vi "FlatToRichcif_manager_CreatePluginLoaderRequest.vi"(5 "OutputClusterType":T1, 11 "InputCluster":T4) -> (3 "OutputCluster":T1)   [LabVIEW 2021, in "CIF_Manager_client.lvlib"]
uses:
  cif_manager_CreatePluginLoaderRequest_Flat.ctl
  cif_manager_LoaderInfo_Flat.ctl
  cif_manager_LoaderType.ctl
  cif_manager_CreatePluginLoaderRequest.ctl
  cif_manager_LoaderInfo.ctl
  CIF_Manager_client.lvlib
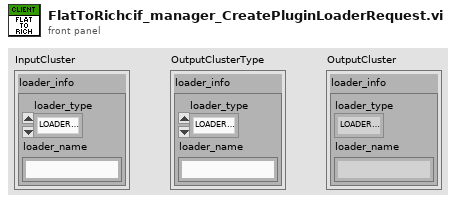
[diagram p1: front panel]
types:
  T1 = typedef "CIF_Manager_client.lvlib/cif_manager_CreatePluginLoaderRequest.ctl" = cluster{"loader_info":T2}
  T2 = typedef "CIF_Manager_client.lvlib/cif_manager_LoaderInfo.ctl" = cluster{"loader_type":T3, "loader_name":string}
  T3 = typedef "CIF_Manager_client.lvlib/cif_manager_LoaderType.ctl" = enum32{"LOADERTYPE_UNKNOWN", "LOADERTYPE_LABVIEW"}
  T4 = typedef "CIF_Manager_client.lvlib/cif_manager_CreatePluginLoaderRequest_Flat.ctl" = cluster{"loader_info":T5}
  T5 = typedef "CIF_Manager_client.lvlib/cif_manager_LoaderInfo_Flat.ctl" = cluster{"loader_type":T3, "loader_name":string}
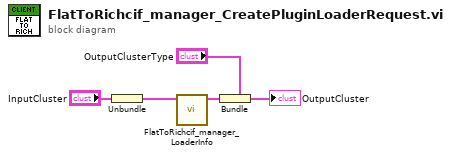
[diagram p0: block diagram]
diagram:
  n1 = Unbundle "Unbundle"("InputCluster") -> ("loader_info"=w2:T5)
  n2 = call "FlatToRichcif_manager_LoaderInfo.vi"("InputCluster"=w2) -> ("OutputCluster"=w1:T2)  [unwired: 10 in]
  n3 = Bundle "Bundle"(cluster="OutputClusterType", "loader_info"=w1) -> (→"OutputCluster":T1)
